vi "GetFileVersion_DotNet.vi"(8 "error in (no error)":errorcluster, 11 "Exe Path":path) -> (0 "error out":errorcluster, 1 "bitness":enum16{"unknown", "32", "64"}(ring), 2 "FileVersion":string, 3 "Exe Path Out":path, 5 "ProductName":string)   [LabVIEW 2017]
doc: "This VI can obtain information about an existing executable, such as its version, product name, and so on, or it can be called as a subVI from a VI that will be built into an executable to obtain information about that executable.\n\nTo obtain version information about an existing executable, enter a path to an executable into Exe Path and run the Vi.\n\nCall this VI as a subVI from a VI that you will build into an executable and leave the path input unwired to obtain the version information about the built executable."
panel:
  # "This VI can obtain information about an\nexisting executable, such as its\nversion, product name, and so on, or it\ncan be called as a subVI from a VI\nthat will be built into an executable to\nobtain information about that\nexecutable.\n\nTo obtain version information about an\nexisting executable, enter a path to an\nexecutable into Exe Path and run the Vi.\n\nCall this VI as a subVI from a VI that\nyou will build into an executable and\nleave the path input unwired to\nobtain the version information about\nthe built executable."
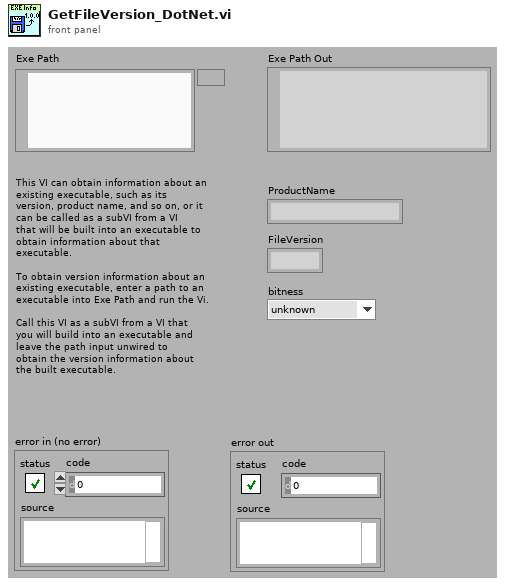
[diagram p1: front panel]
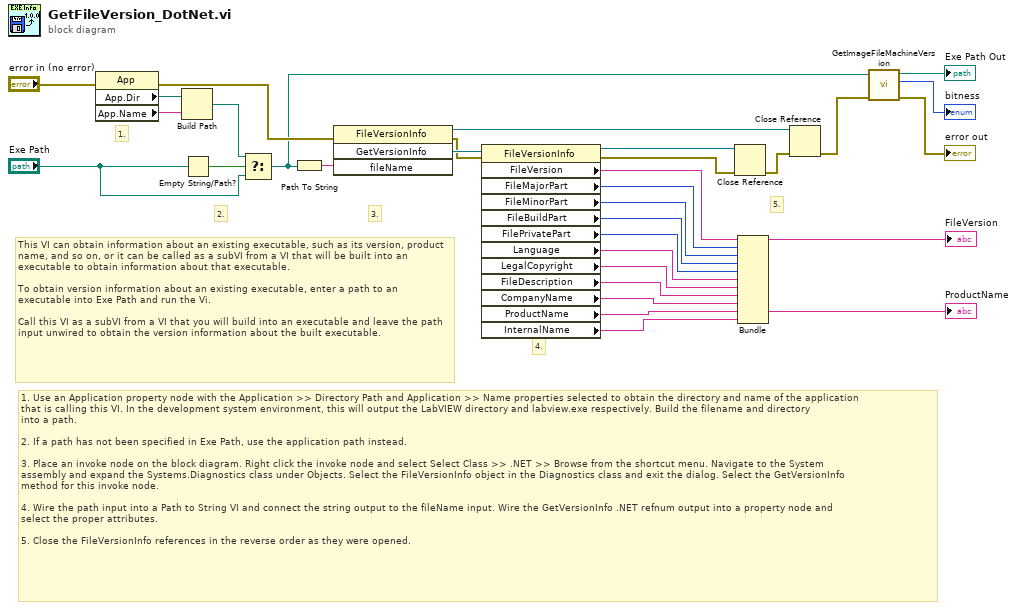
[diagram p0: block diagram]
diagram:
  # "This VI can obtain information about an existing executable, such as its version, product name, and so on, or it can be called as a subVI from a VI that will be built into an executable to obtain information about that executable.\n\nTo obtain version information about an existing executable, enter a path to an executable into Exe Path and run the Vi.\n\nCall this VI as a subVI from a VI that you will build into an executable and leave the path input unwired to obtain the version information about the built executable."
  # "1. Use an Application property node with the Application >> Directory Path and Application >> Name properties selected to obtain the directory and name of the application \nthat is calling this VI. In the development system environment, this will output the LabVIEW directory and labview.exe respectively. Build the filename and directory\ninto a path.\n\n2. If a path has not been specified in Exe Path, use the application path instead.\n\n3. Place an invoke node on the block diagram. Right click the invoke node and select Select Class >> .NET >> Browse from the shortcut menu. Navigate to the System\nassembly and expand the Systems.Diagnostics class under Objects. Select the FileVersionInfo object in the Diagnostics class and exit the dialog. Select the GetVersionInfo\nmethod for this invoke node.\n\n4. Wire the path input into a Path to String VI and connect the string output to the fileName input. Wire the GetVersionInfo .NET refnum output into a property node and\nselect the proper attributes.\n\n5. Close the FileVersionInfo references in the reverse order as they were opened."
  # "5."
  # "4."
  # "1."
  # "3."
  # "2."
  n1 = property class="App"(error in="error in (no error)") -> (error out=w18:errorcluster, "App.Dir"=w25:path, "App.Name"=w24:string)  [unwired: 1 in, 1 out]
  n2 = Build Path(base path=w25, name or relative path=w24) -> (appended path=w21:path)
  n3 = Empty String/Path?(string/path="Exe Path") -> (empty?=w23:bool)
  n4 = Select(t=w21, s=w23, f="Exe Path") -> (s? t:f=w7:path)
  n5 = Path To String(path=w7) -> (string=w28:string)
  n6 = invoke class="FileVersionInfo" method="GetVersionInfo"(error in=w18, "fileName"=w28) -> (reference out=w19:refnum<k24>, error out=w29:errorcluster, "GetVersionInfo"=w30:refnum<k24>)  [unwired: 2 in, 1 out]
  n7 = property class="FileVersionInfo"(reference=w30, error in=w29) -> (reference out=w27:refnum<k24>, error out=w26:errorcluster, "FileVersion"=w1:string, "FileMajorPart"=w16:i32, "FileMinorPart"=w15:i32, "FileBuildPart"=w14:i32, "FilePrivatePart"=w13:i32, "Language"=w12:string, "LegalCopyright"=w11:string, "FileDescription"=w10:string, "CompanyName"=w9:string, "ProductName"=w2:string, "InternalName"=w8:string)
  "FileVersion" <- w1
  "ProductName" <- w2
  n8 = Close Reference(reference=w27, error in (no error)=w26) -> (error out=w20:errorcluster)
  n9 = Bundle("FileVersion"=w1, "FileMajorPart"=w16, "FileMinorPart"=w15, "FileBuildPart"=w14, "FilePrivatePart"=w13, "Language"=w12, "LegalCopyright"=w11, "FileDescription"=w10, "CompanyName"=w9, "ProductName"=w2, "InternalName"=w8) -> ()  [unwired: 1 in, 1 out]
  n10 = Close Reference(reference=w19, error in (no error)=w20) -> (error out=w5:errorcluster)
  n11 = call "GetImageFileMachineVersion.vi"("error in"=w5, "dll Path"=w7) -> ("error out"=→"error out":errorcluster, "bitness"=→"bitness":enum16{"unknown", "32", "64"}, "path"=→"Exe Path Out":path)  [unwired: 7 in]
